vi "mean_nan.vi"(11 "Array":dbl[](array[numeric])) -> (3 "Mean":dbl)   [LabVIEW 2016, in "nan operations.lvlib"]
uses:
  nan operations.lvlib
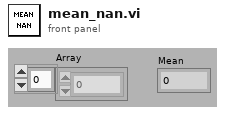
[diagram p1: front panel]
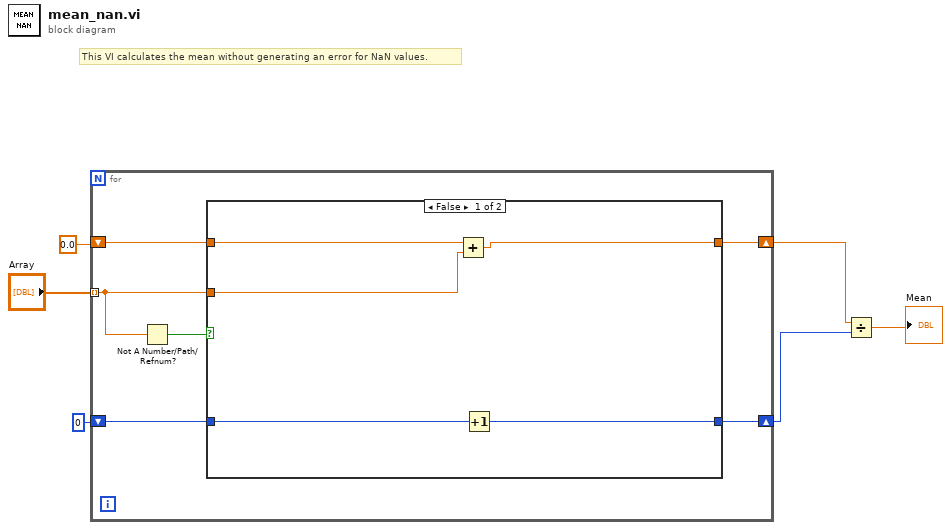
[diagram p0: block diagram]
diagram:
  # "This VI calculates the mean without generating an error for NaN values."
  n1 = for {
    tunnel: "Array" -> [w10] mode=indexing
    shift-right: [w7] -> w2
    shift-left: 0.0 -> [w11]
    shift-right: [w8] -> w1
    shift-left: 0 -> [w9]
    n2 = Not A Number/Path/Refnum?(number/path/refnum=w10) -> (NaN/Path/Refnum?=w12:bool)
    n3 = case shown="False" w12 {
      tunnel: w11 -> [w17 w19]
      tunnel: w10 -> [w16 _]
      tunnel: w9 -> [w15 w18]
      tunnel: [w14 w18] -> w8
      tunnel: [w13 w19] -> w7
      frame False {
        n4 = Add(x=w17, y=w16) -> (x+y=w13:dbl)
        n5 = Increment(x=w15) -> (x+1=w14:i32)
      }
      frame True {
      }
    }
  }
  n6 = Divide(x=w2, y=w1) -> (x/y=→"Mean":dbl)
